vi "FinalizeSubExperiment.vi"(8 "error in (no error)":errorcluster, 9 "repeats":u16=1, 10 "channel":u8, 11 "deviceName":string) -> (0 "error out":errorcluster)   [LabVIEW 2018]
doc: "EXPORT void AisFinalizeSubExperiment(const char* deviceName, uint8_t channel, uint16_t repeats);"
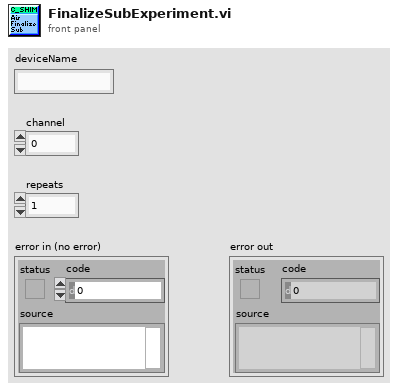
[diagram p1: front panel]
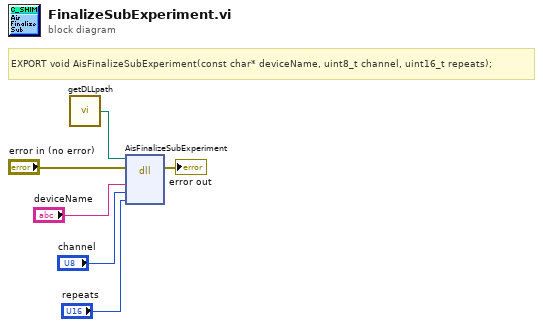
[diagram p0: block diagram]
diagram:
  # "EXPORT void AisFinalizeSubExperiment(const char* deviceName, uint8_t channel, uint16_t repeats);"
  n1 = call "getDLLpath.vi"() -> ("DLL_Path"=w1:path)
  n2 = dll-call lib="?" fn="AisFinalizeSubExperiment"(path in=w1, error in="error in (no error)", "deviceName"="deviceName", "channel"="channel", "repeats"="repeats") -> (error out=→"error out":errorcluster)  [unwired: 5 in, 1 out]
